vi "Invert Numeric.vi"(0 "celing":dbl, 7 "Numeric":dbl, 11 "floor":dbl) -> (4 "coerced(Inverted)":dbl, 8 "Inverted":dbl, 15 "In Range?":bool)   [LabVIEW 2016]
doc: "This VI takes the numeric and inverts it's position on a number line that runs between the floor and celing.\n\nCreated by Team 4130 for use in the 2016-2017 FRC season"
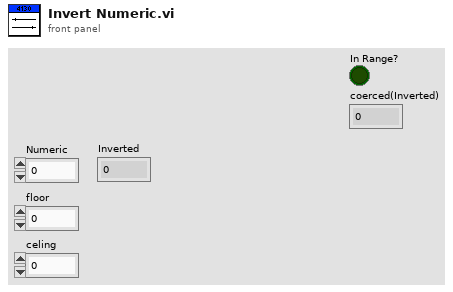
[diagram p1: front panel]
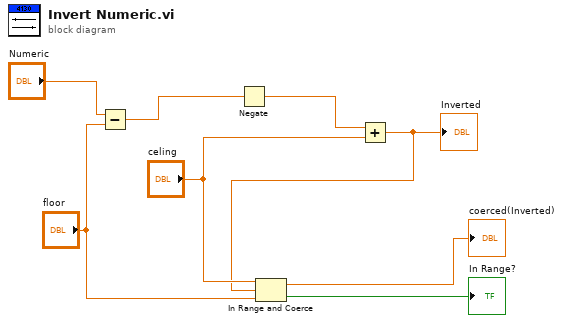
[diagram p0: block diagram]
diagram:
  n1 = Subtract(x="Numeric", y="floor") -> (x-y=w7:dbl)
  n2 = Negate(x=w7) -> (-x=w8:dbl)
  n3 = Add(x=w8, y="celing") -> (x+y=w2:dbl)
  "Inverted" <- w2
  n4 = In Range and Coerce(upper limit="celing", x=w2, lower limit="floor") -> (coerced(x)=→"coerced(Inverted)":dbl, In Range?=→"In Range?":bool)
